vi "VernierCorr.vi"(9 "MINVER":u16, 10 "MAXVER":u16, 11 "Numeric":u16) -> (3 "VernierCorr":i16)   [LabVIEW 2014]
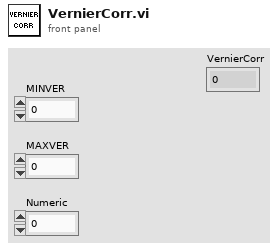
[diagram p1: front panel]
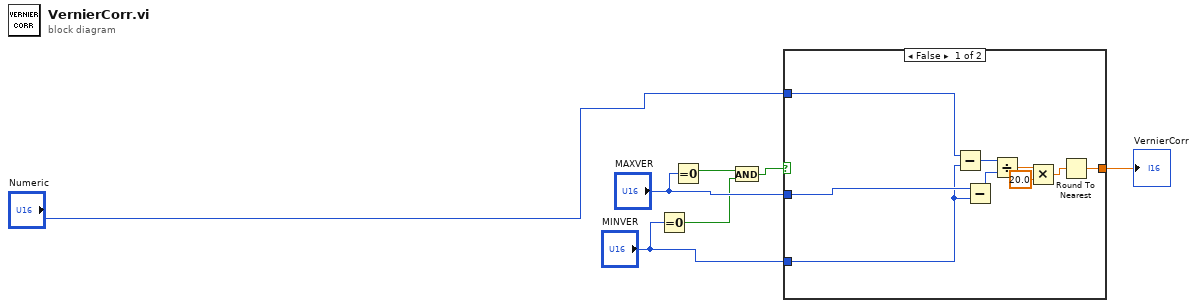
[diagram p0: block diagram]
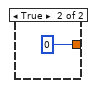
[diagram p2: hidden frame]
diagram:
  n1 = Equal To 0?(x="MINVER") -> (x = 0?=w2:bool)
  n2 = Equal To 0?(x="MAXVER") -> (x = 0?=w3:bool)
  n3 = And(x=w3, y=w2) -> (x .and. y?=w1:bool)
  n4 = case shown="False" w1 {
    tunnel: "MAXVER" -> [w12 _]
    tunnel: "MINVER" -> [w11 _]
    tunnel: "Numeric" -> [w9 _]
    tunnel: [w8 u16 0] -> w6
    frame False {
      n5 = Subtract(x=w9, y=w11) -> (x-y=w10:u16)
      n6 = Subtract(x=w12, y=w11) -> (x-y=w13:u16)
      n7 = Divide(x=w10, y=w13) -> (x/y=w14:sgl)
      n8 = Multiply(x=w14, y=sgl 20.0) -> (x*y=w16:sgl)
      n9 = Round To Nearest(number=w16) -> (nearest integer value=w8:sgl)
    }
    frame True {
    }
  }
  "VernierCorr" <- w6
